vi "Map Master DO to Slave DI for Fixture T-801.vi"(10 "slave device":string="DAQ2", 11 "DO Write Channels (Master)":string[](array[string])=["Targets/Controller/Hardware/Chassis/DAQ/DAQ1/Digital Output/port0/DO0", "Targets/Controller/Hardware/Chassis/DAQ/DAQ1/Digital Output/port0/DO1"]) -> (3 "Map from DO Master to DI Slave":map{string, string}(c390))   [LabVIEW 2020, in "VeriStandTestCase.lvclass"]
doc: "Maps Master AO channels to Slave AI channels for connections made with the T-801 test fixture."
uses:
  VeriStandTestCase.lvclass
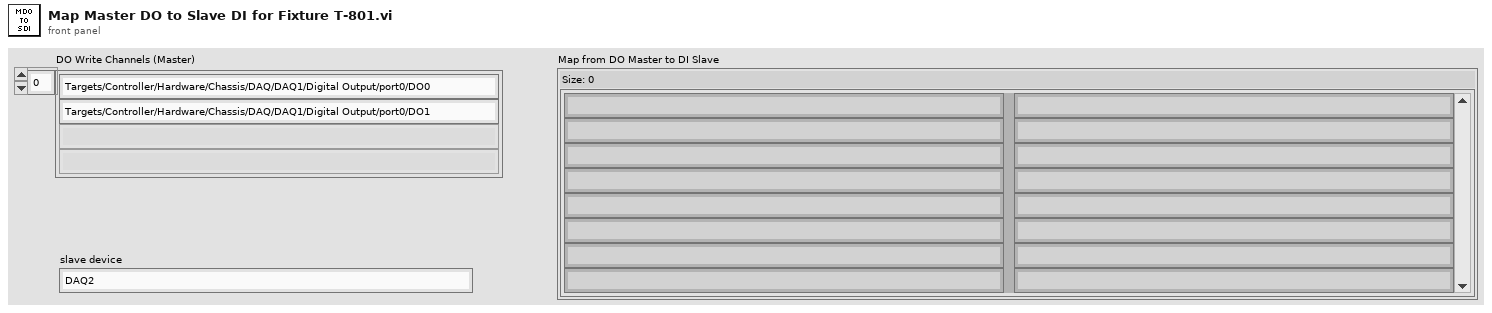
[diagram p1: front panel]
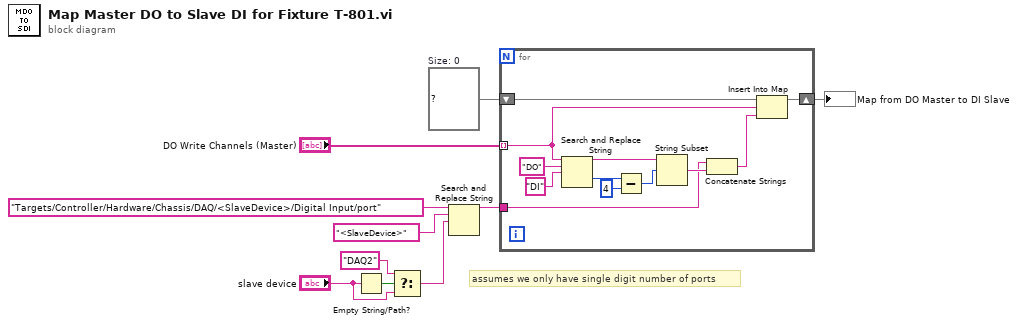
[diagram p0: block diagram]
diagram:
  w3 = map{string, string} {}  # Size: 0
  # "assumes we only have single digit number of ports"
  n1 = Empty String/Path?(string/path="slave device") -> (empty?=w10:bool)
  n2 = Select(t="DAQ2", s=w10, f="slave device") -> (s? t:f=w5:string)
  n3 = Search and Replace String(input string="Targets/Controller/Hardware/Chassis/DAQ/<SlaveDevice>/Digital Input/port", search string="<SlaveDevice>" ("substring (\"\")"), replace string=w5) -> (result string=w2:string)  [unwired: 5 in, 3 out]
  n4 = for {
    tunnel: "DO Write Channels (Master)" -> [w20] mode=indexing
    tunnel: w2 -> [w12]
    shift-right: [w21] -> w1
    shift-left: w3 -> [w22]
    n5 = Search and Replace String(input string=w20, search string="DO", replace string="DI" ("search string")) -> (result string=w15:string, offset past replacement=w17:i32)  [unwired: 5 in, 2 out]
    n6 = Subtract(x=w17, y=4) -> (x-y=w14:i32)
    n7 = String Subset(string=w15, offset (0)=w14) -> (substring=w13:string)  [unwired: 1 in]
    n8 = Concatenate Strings(w12, w13) -> (w11:string)
    n9 = Insert Into Map(map in=w22, key=w20, value=w11) -> (map out=w21:map{string, string})  [unwired: 2 out]
  }
  "Map from DO Master to DI Slave" <- w1
